vi "startsWith.vi"(8 "error in (no error)":errorcluster, 11 "CommandProcessor in":refnum<class "CommandProcessor.lvclass">) -> (0 "error out":errorcluster, 1 "element":string, 2 "command":string, 3 "CommandProcessor out":refnum<class "CommandProcessor.lvclass">)   [LabVIEW 2011, in "Tools.lvlib" / "Interpreters.lvlib" / "CommandProcessor.lvclass"]
uses:
  CommandProcessor.lvclass
  CommandProcessor.lvclass/CommandProcessor.ctl
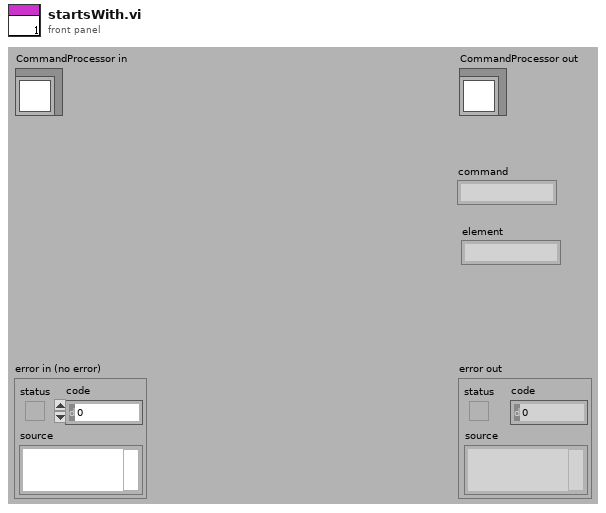
[diagram p1: front panel]
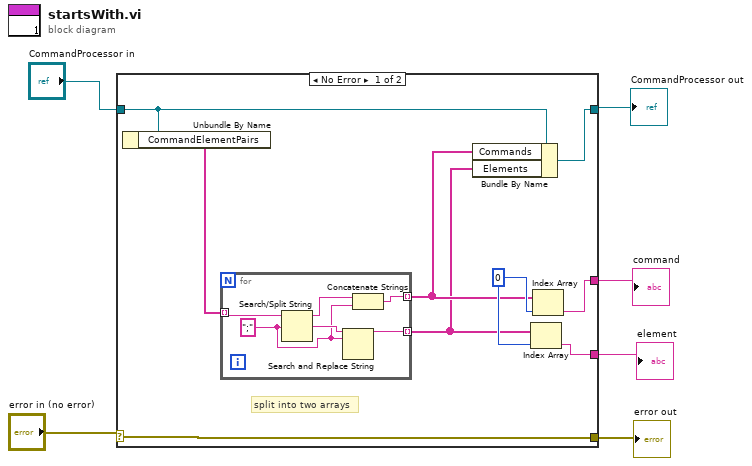
[diagram p0: block diagram]
diagram:
  n1 = case shown="No Error" "error in (no error)" {
    selector: "error in (no error)" -> [w14 w23]
    tunnel: [w14 w23] -> w5
    tunnel: [w9 w22] -> w3
    tunnel: "CommandProcessor in" -> [w10 w22]
    tunnel: [w12 _] -> w2
    tunnel: [w11 _] -> w1
    frame No Error {
      w13 = 0
      # "split into two arrays"
      n2 = Unbundle By Name(w10) -> ("CommandElementPairs"=w15:string[])
      n3 = for {
        tunnel: w15 -> [w21] mode=indexing
        tunnel: [w18] -> w8 mode=indexing
        tunnel: [w19] -> w7 mode=indexing
        w16 = ";"
        n4 = Search/Split String(string=w21, search string/char (-)=w16) -> (substring before match=w17:string, match + rest of string=w20:string)  [unwired: 1 in, 1 out]
        n5 = Search and Replace String(input string=w20, search string=w16) -> (result string=w19:string)  [unwired: 6 in, 3 out]
        n6 = Concatenate Strings(w17, w16) -> (w18:string)
      }
      n7 = Bundle By Name(cluster=w10, "Commands"=w8, "Elements"=w7) -> (w9:refnum<class "CommandProcessor.lvclass">)
      n8 = Index Array(array=w7, index=w13) -> (element=w11:string)
      n9 = Index Array(array=w8, index=w13) -> (element=w12:string)
    }
    frame Error {
    }
  }
  "error out" <- w5
  "CommandProcessor out" <- w3
  "command" <- w2
  "element" <- w1
